vi "LogDBBoolChangeArray.vi"(4 "db connection":bool, 5 "names":string[](array[string]), 6 "cluster reading time":timestamp, 7 "prefix":string, 8 "error in (no error)":errorcluster, 9 "shift reg in":bool[](array[boolean]), 10 "values":bool[](array[boolean]), 11 "db reference":T1) -> (0 "error out":errorcluster, 1 "shift reg out":bool[](array[boolean]), 2 "db connection":bool, 3 "db reference out":T1)   [LabVIEW 2011]
uses:
  <vilib>/addons/database/Connection.llb/Conn ObjectReference.ctl
  <vilib>/Utility/error.llb/DialogType.ctl
  <vilib>/addons/database/NI_Database_API.lvlib
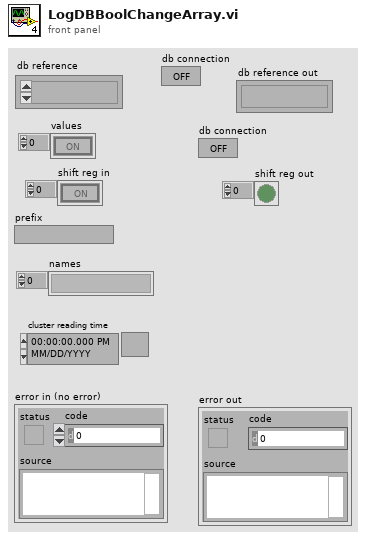
[diagram p1: front panel]
types:
  T1 = typedef "NI_Database_API.lvlib/Conn ObjectReference.ctl" = refnum<k1>
  T2 = typedef "DialogType.ctl" = u16
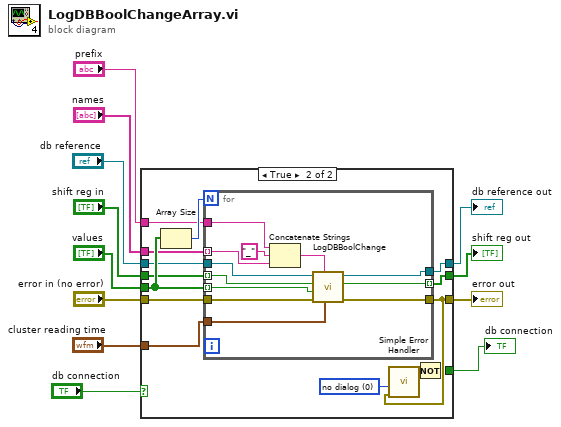
[diagram p0: block diagram]
diagram:
  n1 = case shown="True" "db connection" {
    selector: "db connection" -> [w13 _]
    tunnel: "error in (no error)" -> [w16 w30]
    tunnel: [w15 w29] -> w11
    tunnel: "values" -> [_ w27]
    tunnel: "names" -> [_ w26]
    tunnel: "shift reg in" -> [w15 w25]
    tunnel: "db reference" -> [w14 w24]
    tunnel: "prefix" -> [_ w23]
    tunnel: "cluster reading time" -> [_ w22]
    tunnel: [w14 w21] -> w4
    tunnel: [w16 w20] -> w3
    tunnel: [w13 w17] -> w1
    frame False {
    }
    frame True {
      w18 = T2 0 items=["no dialog", "OK message", "continue or stop message", "OK message + warnings", "continue/stop + warnings"] ("type of dialog (OK msg:1)")
      n2 = Array Size(array=w27) -> (size(s)=w28:i32)
      n3 = for {
        N: w28 -> [_]
        tunnel: w23 -> [w42]
        tunnel: w26 -> [w39] mode=indexing
        tunnel: [w38] -> w21
        tunnel: [w37] -> w20
        tunnel: w30 -> [w36]
        tunnel: w22 -> [w34]
        tunnel: [w35] -> w29 mode=indexing
        tunnel: w24 -> [w33]
        tunnel: w25 -> [w32] mode=indexing
        tunnel: w27 -> [w31] mode=indexing
        n4 = Concatenate Strings(w42, "_" ("string"), w39) -> (w40:string)
        n5 = call "LogDBBoolChange.vi"("current time"=w34, "db table name"=w40, "error in"=w36, "value"=w31, "shiftReg"=w32, "Refnum in"=w33) -> ("error out"=w37:errorcluster, "shiftReg"=w35:bool, "Refnum out"=w38:T1)  [unwired: 3 in]
      }
      n6 = call <vilib>:"Simple Error Handler.vi"("type of dialog (OK msg:1)"=w18, "error in (no error)"=w20) -> ("error?"=w19:bool)  [unwired: 3 in, 4 out]
      n7 = Not(x=w19) -> (.not. x?=w17:bool)
    }
  }
  "shift reg out" <- w11
  "db reference out" <- w4
  "error out" <- w3
  "db connection" <- w1
